vi "ICM Open Parser.vi"(8 "error in (no error)":errorcluster, 11 "ICM File In":path) -> (0 "error out":errorcluster, 3 "Parser out":refnum<class "Parser.lvclass">)   [LabVIEW 2015]
doc: "ICM Open Parser.vi\n\nThis VI finds the Parser of the current configuration file, opens the object, and reads its configuration data.\n\nInstrument Communication Module Version 1.0\nSeptember, 2017 Original Code Consulting David Thomson\n www.originalcode.com"
uses:
  Parser/Parser.lvclass
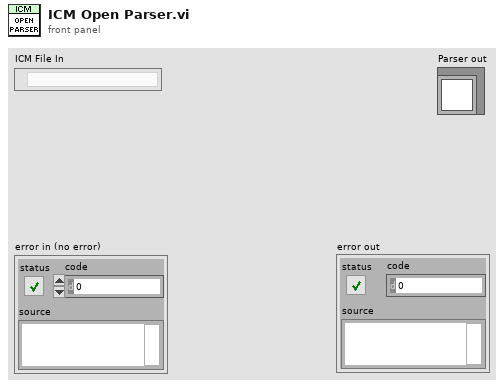
[diagram p1: front panel]
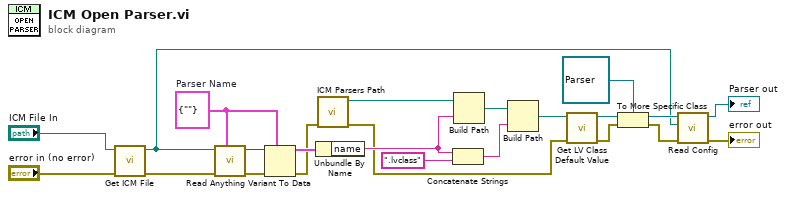
[diagram p0: block diagram]
diagram:
  w21 = cluster{"name":string} {"name"=""}  # Parser Name
  n1 = call "Get ICM File.vi"("error in (no error)"="error in (no error)", "ICM File In"="ICM File In") -> ("error out"=w7:errorcluster, "ICM File"=w4:path)  [unwired: 8 in]
  n2 = call "Read Anything.vi"("Type of Anything"=w21, "Error In"=w7, "Path (dialog)"=w4) -> ("Error Out"=w23:errorcluster, "Anything"=w22:variant)  [unwired: 6 in, 1 out]
  n3 = Variant To Data(error in=w23, type=w21, Variant=w22) -> (data=w16:cluster{"name":string}, error out=w2:errorcluster)
  n4 = Unbundle By Name(w16) -> ("name"=w15:string)
  n5 = call "ICM Parsers Path.vi"("error in (no error)"=w2) -> ("error out"=w1:errorcluster, "ICM Parsers Path"=w3:path)  [unwired: 9 in]
  n6 = Concatenate Strings(w15, ".lvclass" ("string")) -> (w17:string)
  n7 = Build Path(base path=w3, name or relative path=w15) -> (appended path=w19:path)
  n8 = Build Path(base path=w19, name or relative path=w17) -> (appended path=w20:path)
  n9 = call <vilib>:"Get LV Class Default Value.vi"("error in (no error)"=w1, "class path"=w20) -> ("error out"=w14:errorcluster, "object"=w13:refnum<class>)  [unwired: 8 in]
  n10 = To More Specific Class(target class=refnum<class "Parser.lvclass"> refnum ("Parser.lvclass"), reference=w13, error in=w14) -> (specific class reference=w11:refnum<class "Parser.lvclass">, error out=w10:errorcluster)
  n11 = call-dynamic "Read Config.vi"("error in (no error)"=w10, "ICM File In"=w4, "Parser in"=w11) -> ("error out"=→"error out":errorcluster, "Parser out"=→"Parser out":refnum<class "Parser.lvclass">)  [unwired: 7 in]
